vi "Main Loop.vi"(8 "error in (no error)":errorcluster, 10 "Chart Notifier":refnum<notifier>, 11 "Message Queues":T1) -> (0 "error out":errorcluster)   [LabVIEW 2018, in "TCU Module.lvlib" / "TCU Module Engine.lvlib"]
uses:
  TCU Module Engine.lvlib
  All Message Queues.ctl
  support/Message Queue/Message Cluster.ctl
  TCU State Cluster.ctl
  State Enum.ctl
  TCU Module Settings Cluster.ctl
  Output Devices.ctl
  Huber TCU/Huber Settings.ctl
  Lauda Integral XT-150 TCU/Lauda Settings.ctl
  Julabo Type 1 TCU/Julabo Type 1 TCU Folder/Julabo FP-50 Settings.ctl
  Huber Unistat 410 TCU/Huber Unistat 410 RS485 Settings.ctl
  TCU Module Display.ctl
  <vilib>/Platform/TimedLoop/XDataNode/timing_clust.ctl
  <vilib>/Platform/TimedLoop/XDataNode/nitl_modes.ctl
  <vilib>/Platform/TimedLoop/XDataNode/wakeup.ctl
  Tag VIs/Tag FGV Operation Enum.ctl
  TCU Module Config Cluster.ctl
  <vilib>/Utility/miscctls.llb/LVPoint32TypeDef.ctl
  support/Message Queue/Enqueue Message (Single).vi
  <vilib>/Platform/TimedLoop/XDataNode/XDataNode.xnode
  support/Message Queue/Message Queue.lvlib
  <vilib>/Platform/TimedLoop/XDataNode/XDNodeRunTimeDep.lvlib
  TCU Module.lvlib
  Shared Variables/Dynamic Shared Variables.lvlib
  Huber TCU/Huber Ministat 230 TCU.lvlib
  Lauda Integral XT-150 TCU/Lauda TCU.lvlib
  Julabo Type 1 TCU/Julabo Type 1 TCU Folder/Julabo Type FP-50 TCU.lvlib
  support/Support Library.lvlib
  Huber Unistat 410 TCU/Huber Unistat 410 TCU.lvlib
panel:
  out "Period (s)":dbl format="%_4g"
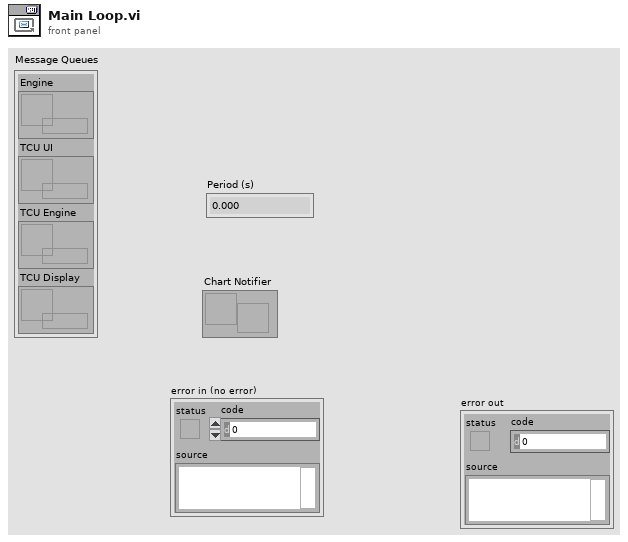
[diagram p1: front panel]
types:
  T1 = typedef "TCU Module.lvlib/All Message Queues.ctl" = cluster{"Engine":refnum<queue>, "TCU UI":refnum<queue>, "TCU Engine":refnum<queue>, "TCU Display":refnum<queue>}
  T2 = typedef "XDNodeRunTimeDep.lvlib/timing_clust.ctl" = cluster{"Expected End [f-1]":u64, "Actual End [f-1]":u64, "Finished Late? [f-1]":bool, "Expected End [i-1]":u64, "Actual End [i-1]":u64, "Finished Late? [i-1]":bool, "Expected Start [i]":u64, "Actual Start [i]":u64, "Expected Start [f]":u64, "Actual Start [f]":u64, "Source Name":string, "Structure Name":string, "Period":i64, "Deadline":i64, "Offset":i64, "Start":i64, "Priority":i32, "Timeout":i32, "Mode":T3, "Wakeup Reason":T4, "Error":errorcluster, "Source Type":string, "Secondary Source Type":string, "Global End Time":u64, "Global Start Time":u64, "Frame Duration":u64, "Iteration Duration":u64, "Assigned CPU":i32, "I/O Scan Engine Mode":u32}
  T3 = typedef "XDNodeRunTimeDep.lvlib/nitl_modes.ctl" = enum32{"No Change", "Process missed periods, maintain original phase", "Discard missed periods, maintain original phase", "Process missed periods, ignore original phase", "Discard missed periods, ignore original phase"}
  T4 = typedef "XDNodeRunTimeDep.lvlib/wakeup.ctl" = enum32{"Normal", "Aborted", "Asynchronous wakeup", "Timing source error", "Timed loop error", "Timeout"}
  T5 = cluster{"enable? (F)":bool, "name":string, "alarm on":bool, "priority":u32, "ack type":enum16{"Auto", "User", "None", "Each Occurrence"}, "area":string, "description":string, "log? (T)":bool}
  T6 = typedef "Tag FGV Operation Enum.ctl" = enum16{"Init", "Set Notification Queue", "Create Tag", "Commit", "Write Tag (Numeric)", "Write Tag (Boolean)", "Read All Tags", "Read One Tag", "Delete Tag Category", "Set Alarm Parameters (Numeric)", "Set Alarm Parameters (Boolean)", "Enable All Alarms", "Disable All Alarms", "Delete All Tags", "Read Alarms", "Ack Alarm", "Read Alarm Parameters (Numeric)", "Read Alarm Parameters (Boolean)"}
  T7 = enum32{"u32BitField", "bool", "double", "string", "int8", "uint8", "int16", "uint16", "int32", "uint32", "int64", "uint64", "single", "double waveform", "int16 waveform", "array of boolean", "array of int8", "array of uint8", "array of int16", "array of uint16", "array of int32", "array of uint32", "array of int64", "array of uint64", "array of single", "array of double", "array of double waveform", "array of int16 waveform", "array of string", "variant", "timestamp", "fixed point", "custom"}
  T8 = typedef "TCU Module.lvlib/TCU Module Engine.lvlib/State Enum.ctl" = enum16{"Measuring", "Idle", "Paused"}
  T9 = typedef "TCU Module.lvlib/TCU Module Config Cluster.ctl" = cluster{"GUID":string, "Drop Coords":T10, "Process Name":string, "User name":string, "Queue Name":string, "Settings":T11, "Load Count":i32, "Power Level Changed":bool}
  T10 = typedef "LVPoint32TypeDef.ctl" = cluster{"Horizontal":i32, "Vertical":i32}
  T11 = typedef "TCU Module.lvlib/TCU Module Settings Cluster.ctl" = cluster{"Cycle Period":dbl, "Setpoint Entry":dbl, "Output Device":T12, "Huber Ministat 230 Settings":T13, "Lauda Settings":T14, "Julabo FP-50 Settings":T15, "Internal Control?":bool, "Huber Unistat 410 Settings":T16}
  T12 = typedef "Output Devices.ctl" = enum16{"Default", "Huber Ministat 230", "Huber Unistat 410", "Lauda XT-150", "Julabo FP-50"}
  T13 = typedef "Huber Ministat 230 TCU.lvlib/Huber Settings.ctl" = cluster{"VISA resource name":refnum<visa-resource-name>, "Simulated?":bool}
  T14 = typedef "Lauda TCU.lvlib/Lauda Settings.ctl" = cluster{"VISA resource name":refnum<visa-resource-name>, "Simulated?":bool, "Pump Power":i32}
  T15 = typedef "Julabo Type FP-50 TCU.lvlib/Julabo FP-50 Settings.ctl" = cluster{"VISA resource name":refnum<visa-resource-name>, "Simulated?":bool, "Pump Power":i32}
  T16 = typedef "Huber Unistat 410 TCU.lvlib/Huber Unistat 410 RS485 Settings.ctl" = cluster{"VISA resource name":refnum<visa-resource-name>, "Address":i8, "Simulated?":bool}
  T17 = typedef "TCU Module.lvlib/TCU Module Display.ctl" = cluster{"TCU On?":bool, "Cycle Period":dbl, "Current TCU Temp":dbl}
  T18 = typedef "TCU Module.lvlib/TCU Module Engine.lvlib/TCU State Cluster.ctl" = cluster{"State":T8, "Start Time":timestamp, "Configuration":T11, "Current Time":timestamp, "First Iteration":bool, "Data":cluster{"TCU Speed":dbl, "Temperature":dbl}, "Process Name":string, "TCU On?":bool, "Output Error":bool, "Start Log":bool, "Power Level Changed":bool}
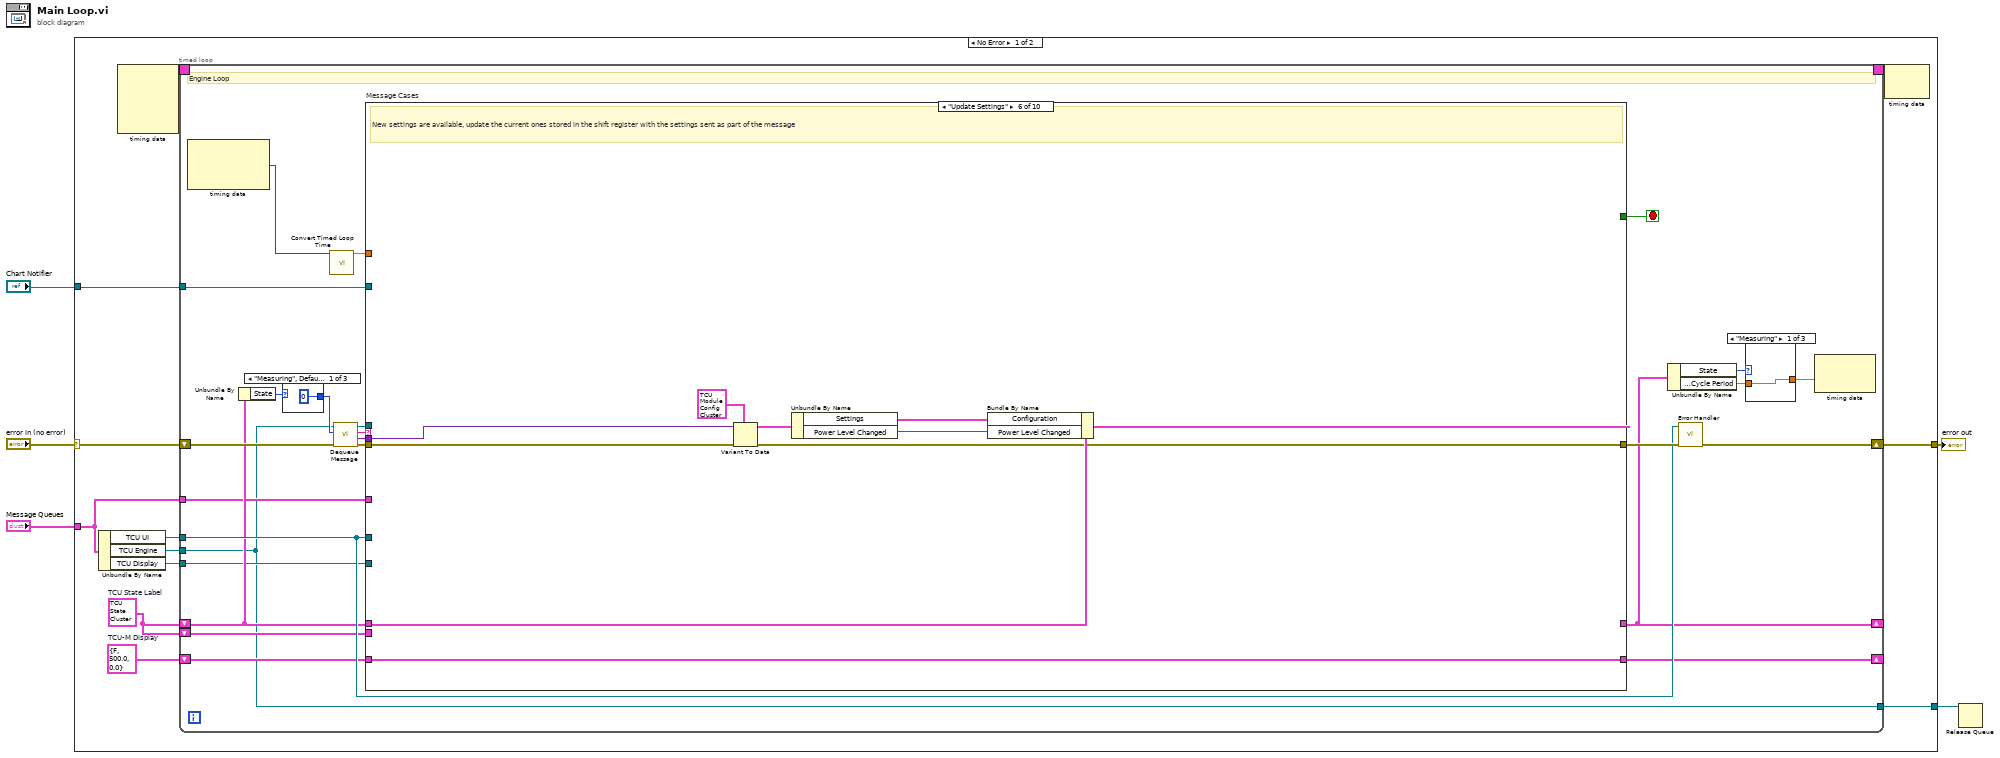
[diagram p0: block diagram]
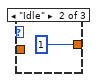
[diagram p2: hidden frame]
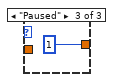
[diagram p3: hidden frame]
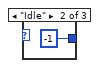
[diagram p4: hidden frame]
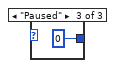
[diagram p5: hidden frame]
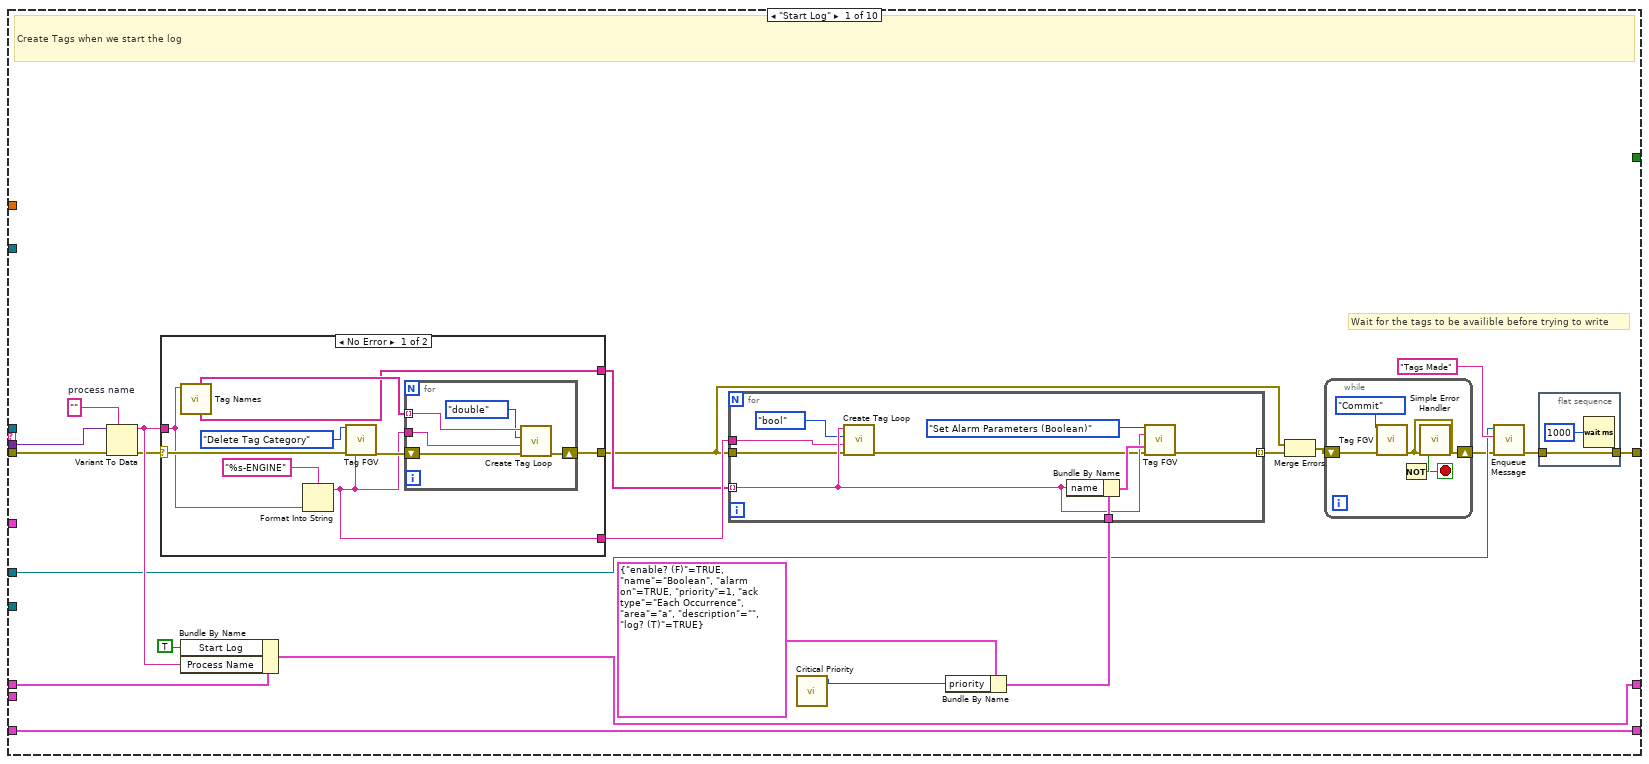
[diagram p6: hidden frame]
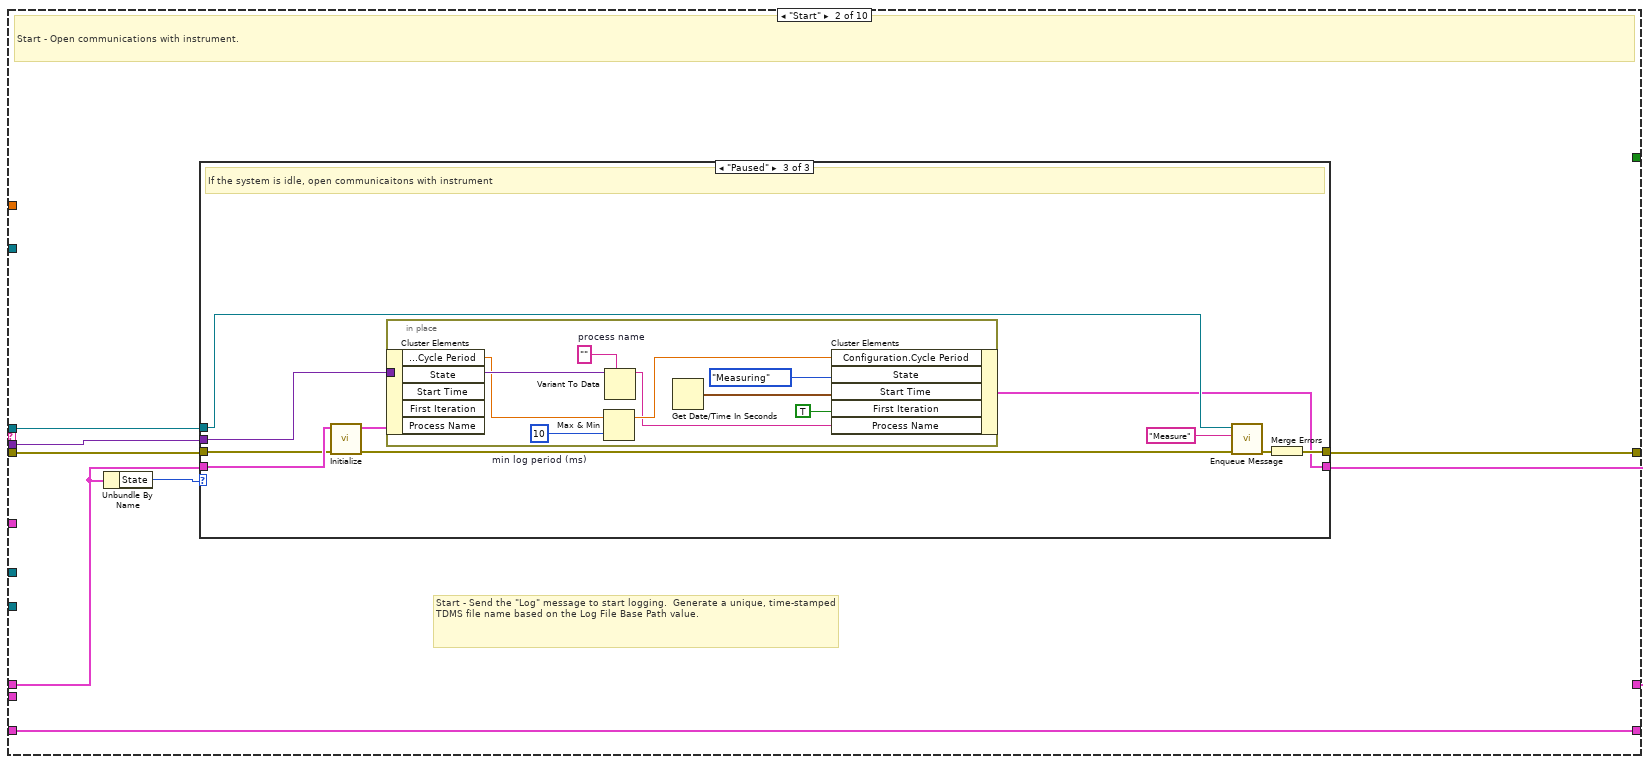
[diagram p8: hidden frame]
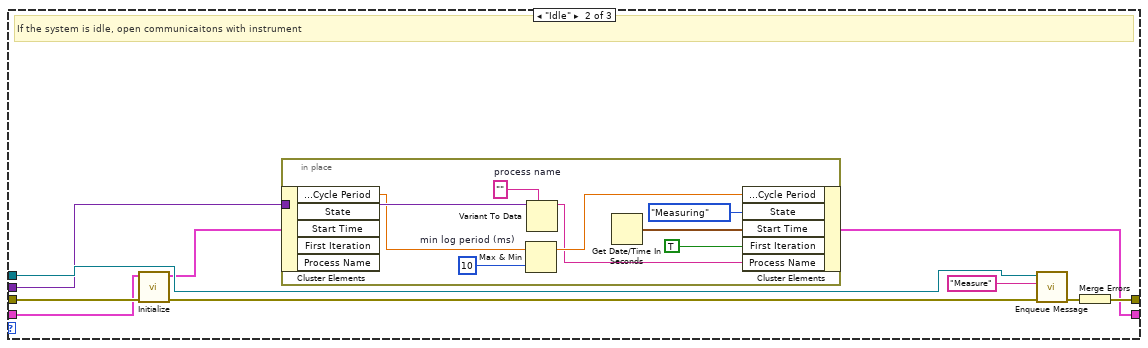
[diagram p10: hidden frame]
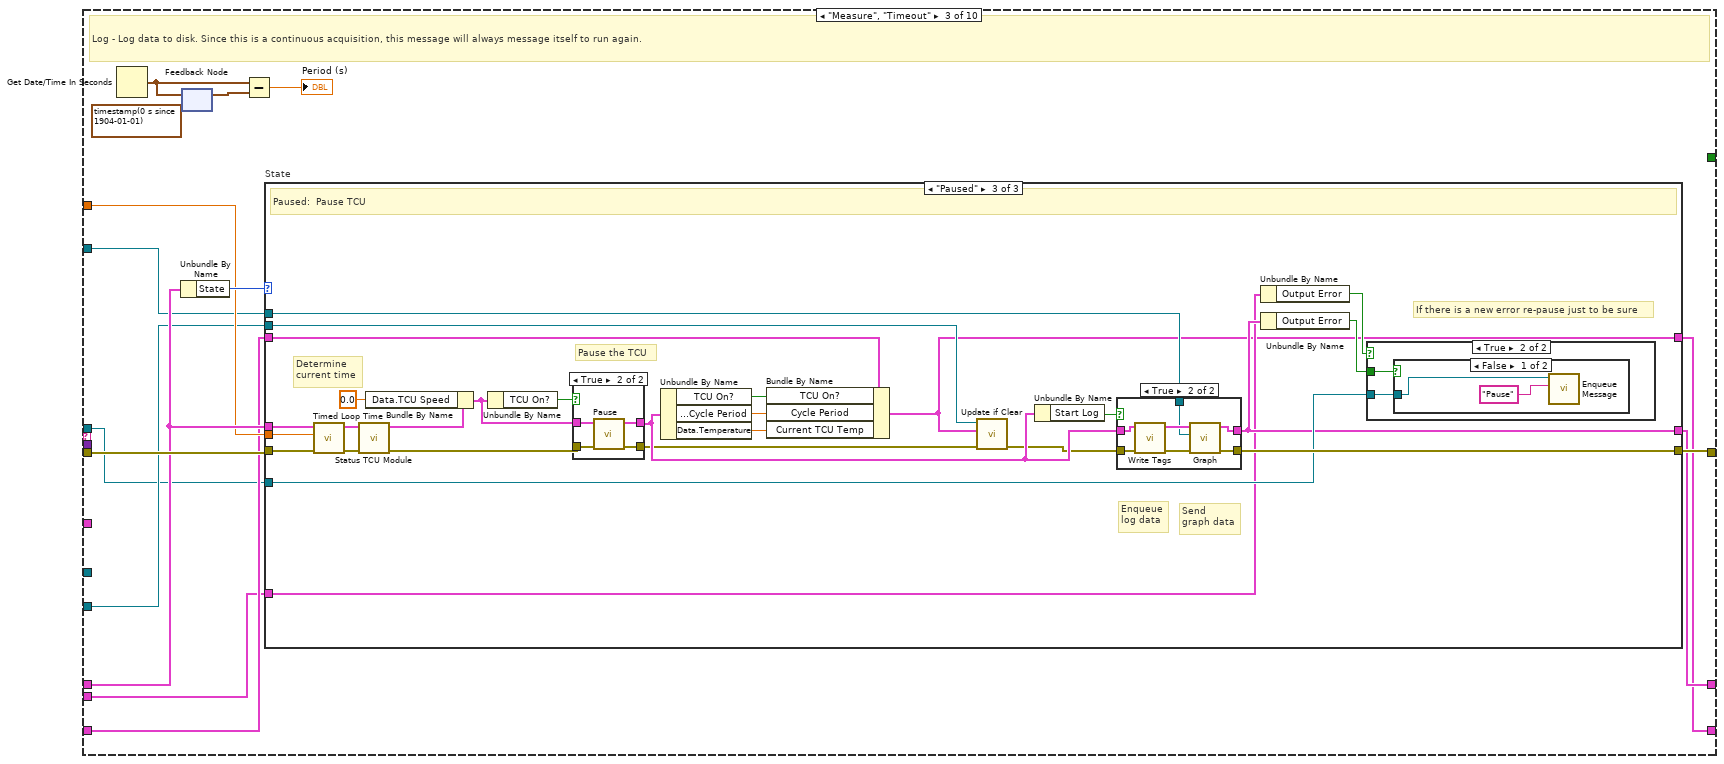
[diagram p11: hidden frame]
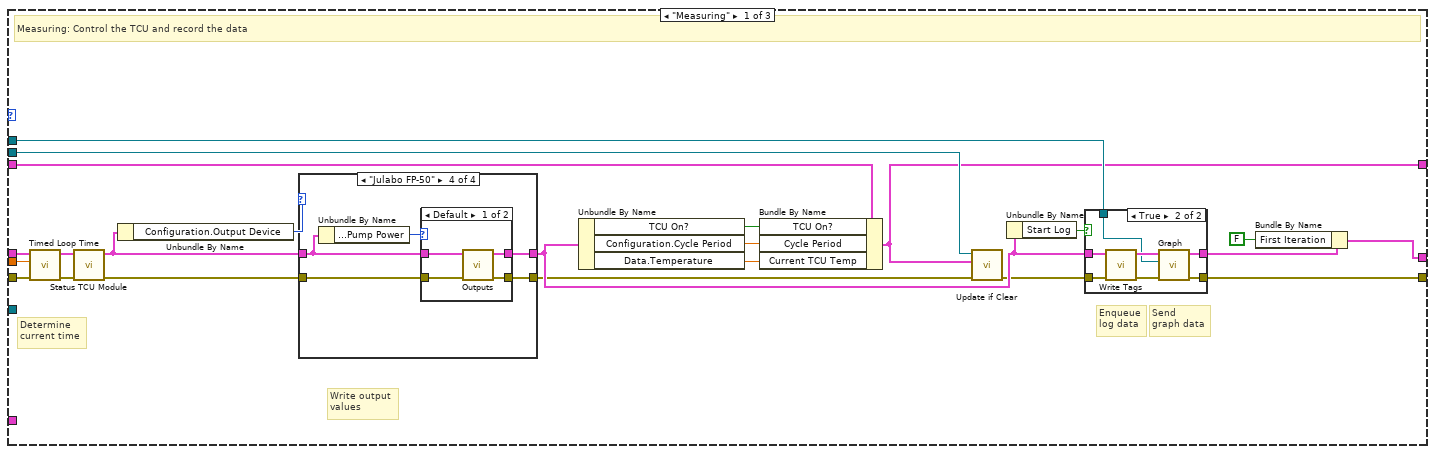
[diagram p12: hidden frame]
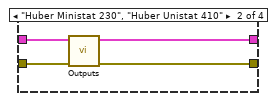
[diagram p14: hidden frame]
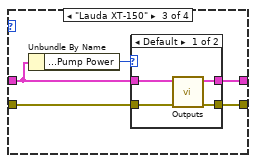
[diagram p15: hidden frame]
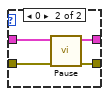
[diagram p16: hidden frame]
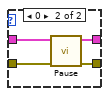
[diagram p17: hidden frame]
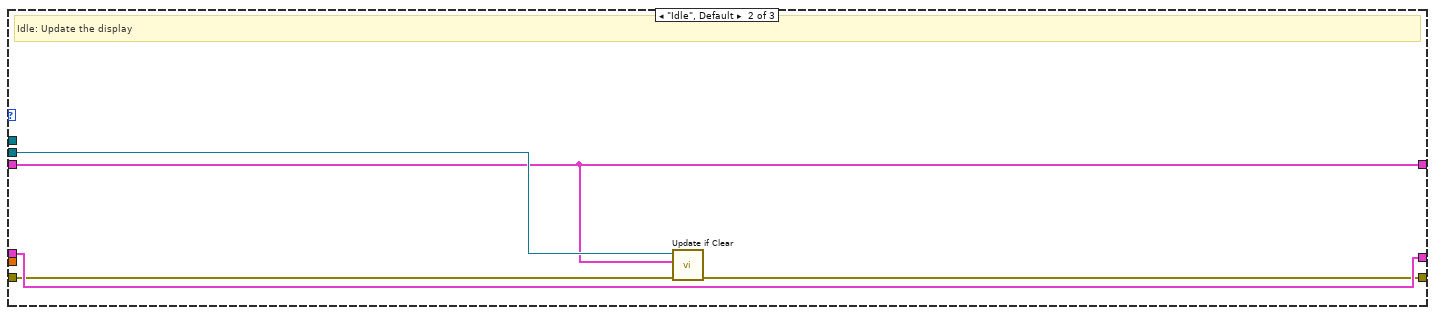
[diagram p19: hidden frame]
diagram:
  n1 = case shown="No Error" "error in (no error)" {
    selector: "error in (no error)" -> [w16 w370]
    tunnel: "Message Queues" -> [w12 _]
    tunnel: [w17 w370] -> w4
    tunnel: "Chart Notifier" -> [w10 _]
    tunnel: [w6 _] -> w1
    frame No Error {
      w8 = T17 {"TCU On?"=FALSE, "Cycle Period"=500.0, "Current TCU Temp"=0.0}  # TCU-M Display
      w7 = T18 {"State"=enum."Idle", "Start Time"=timestamp(0 s since 1904-01-01), "Configuration"={"Cycle Period"=0.0, "Setpoint Entry"=0.0, "Output Device"=enum."Default", "Huber Ministat 230 Settings"={"VISA resource name"="", "Simulated?"=FALSE}, "Lauda Settings"={"VISA resource name"="", "Simulated?"=FALSE, "Pump Power"=2}, "Julabo FP-50 Settings"={"VISA resource name"="", "Simulated?"=FALSE, "Pump Power"=2}, "Internal Control?"=FALSE, "Huber Unistat 410 Settings"={"VISA resource name"="", "Address"=0, "Simulated?"=FALSE}}, "Current Time"=timestamp(0 s since 1904-01-01), "First Iteration"=FALSE, "Data"={"TCU Speed"=0.0, "Temperature"=0.0}, "Process Name"="", "TCU On?"=FALSE, "Output Error"=FALSE, "Start Log"=FALSE, "Power Level Changed"=FALSE}  # TCU State Label
      n2 = Unbundle By Name(w12) -> ("TCU UI"=w15:refnum<queue>, "TCU Engine"=w11:refnum<queue>, "TCU Display"=w9:refnum<queue>)
      n3 = node-c288() -> (w14:T2)  [unwired: 4 in]
      n4 = timed-loop {
        tunnel: w11 -> [w18]
        shift-right: [w30] -> _
        shift-left: w7 -> [w33]
        shift-right: [w35] -> w17
        shift-left: w16 -> [w41]
        tunnel: w15 -> [w34]
        timing: w14 -> [_]
        timing-out: [_] -> w13
        tunnel: w12 -> [w24]
        tunnel: w10 -> [w23]
        tunnel: w9 -> [w22]
        shift-right: [w21] -> _
        shift-left: w8 -> [w20]
        shift-left: w7 -> [w19]
        tunnel: [w18] -> w6
        stop <- w42 stop-if-true
        # "Engine Loop"
        n5 = node-c288() -> (w26:i64)  [unwired: 1 in, 2 out]
        n6 = Unbundle By Name(w33) -> ("State"=w32:T8)
        n7 = case shown="\"Measuring\", Default" w32 {
          tunnel: [0 ("timeout in ms (-1)") -1 ("timeout in ms (-1)") 0 ("timeout in ms (-1)")] -> w31
          frame "Measuring", Default {
          }
          frame "Idle" {
          }
          frame "Paused" {
          }
        }
        n8 = call "Convert Timed Loop Time.vi"("Actual Start [i]"=w26) -> ("ET since start (s)"=w25:dbl)  [unwired: 10 in]
        n9 = call "Dequeue Message.vi"("error in (no error)"=w41, "timeout in ms (-1)"=w31, "Message Queue"=w18) -> ("error out"=w40:errorcluster, "Message Data"=w38:variant, "Message"=w39:string, "dup Message Queue"=w37:refnum<queue>)  [unwired: 5 in]
        n10 = case "Message Cases" shown="\"Update Settings\"" w39 {
          selector: w39 -> [_ _ _ _ _ _ _ _ _ w360]
          tunnel: w37 -> [_ w113 w157 _ _ _ w342 _ _ _]
          tunnel: w40 -> [w73 w112 w168 w294 w313 w336 w345 w352 w359 _]
          tunnel: [w55 w114 w169 w286 w306 w332 w347 w350 w358 w361] -> w36
          tunnel: w33 -> [w72 w108 w166 w291 w311 w334 w340 w351 w356 w367]
          tunnel: [w71 w111 w167 w290 w310 w333 w340 w351 w353 w367] -> w30
          tunnel: [_ _ _ _ _ _ TRUE _ _ _] -> w42
          tunnel: w38 -> [w74 w109 _ _ _ w337 _ _ _ _]
          tunnel: w34 -> [w59 _ _ w293 _ _ w346 _ _ _]
          tunnel: w25 -> [_ _ w165 _ _ _ _ _ _ _]
          tunnel: w24 -> [_ _ _ _ _ _ _ _ _ _]
          tunnel: w23 -> [_ _ w161 _ _ _ _ _ _ _]
          tunnel: w22 -> [_ _ w160 w289 w309 _ _ _ _ _]
          tunnel: w20 -> [w75 w107 w159 w288 w308 w335 w338 w349 w357 w366]
          tunnel: [w75 w107 w158 w288 w308 w335 w338 w349 w357 w366] -> w21
          tunnel: w19 -> [_ _ w156 _ _ _ _ _ _ _]
          frame "Start Log" {
            w70 = ""  # process name
            # "Wait for the tags to be availible before trying to write"
            # "Create Tags when we start the log"
            n11 = Variant To Data(error in=w73, type=w70, Variant=w74) -> (data=w69:string, error out=w68:errorcluster)
            n12 = case shown="No Error" w68 {
              selector: w68 -> [w97 w106]
              tunnel: [w100 w106] -> w54
              tunnel: w69 -> [w95 _]
              tunnel: [w93 _] -> w64
              tunnel: [w92 _] -> w63
              frame No Error {
                n13 = call "Tag Names.vi"("Process Name"=w95) -> ("All Boolean Tags"=w92:string[], "All  Numeric Tags"=w94:string[])  [unwired: 8 in, 1 out]
                n14 = Format Into String(format string="%s-ENGINE", w95) -> (resulting string=w93:string)  [unwired: 2 in, 1 out]
                n15 = call "Tag FGV.vi"("Operation"=Tag_FGV_Operation_Enum."Delete Tag Category", "error in (no error)"=w97, "Tag Category"=w93) -> ("error out"=w96:errorcluster)  [unwired: 5 in, 7 out]
                n16 = for {
                  shift-right: [w101] -> w100
                  shift-left: w96 -> [w104]
                  tunnel: w93 -> [w103]
                  tunnel: w94 -> [w105] mode=indexing
                  n17 = call "Create Tag Loop.vi"("error in (no error)"=w104, "Tag Category"=w103, "data type"=T7."double", "Tag Name"=w105) -> ("error out"=w101:errorcluster)  [unwired: 7 in]
                }
              }
              frame Error {
              }
            }
            n18 = Bundle By Name(cluster=w72, "Start Log"=TRUE, "Process Name"=w69) -> (w71:T18)
            n19 = call "Critical Priority.vi"() -> ("critical priority"=w67:i32)  [unwired: 11 in]
            n20 = Bundle By Name(cluster=T5 {"enable? (F)"=TRUE, "name"="Boolean", "alarm on"=TRUE, "priority"=1, "ack type"=enum."Each Occurrence", "area"="a", "description"="", "log? (T)"=TRUE} ("Boolean alarm settings"), "priority"=w67) -> (w65:T5)
            n21 = for {
              tunnel: w65 -> [w91]
              tunnel: [w90] -> w62 mode=indexing
              tunnel: w63 -> [w87] mode=indexing
              tunnel: w54 -> [w84]
              tunnel: w64 -> [w85]
              n22 = call "Create Tag Loop.vi"("error in (no error)"=w84, "Tag Category"=w85, "data type"=T7."bool", "Tag Name"=w87) -> ("error out"=w83:errorcluster)  [unwired: 7 in]
              n23 = Bundle By Name(cluster=w91, "name"=w87) -> (w89:T5)
              n24 = call "Tag FGV.vi"("Operation"=Tag_FGV_Operation_Enum."Set Alarm Parameters (Boolean)", "Tag Name"=w87, "Data"=w89, "error in (no error)"=w83) -> ("error out"=w90:errorcluster)  [unwired: 4 in, 7 out]
            }
            n25 = Merge Errors(w54, w62) -> (w58:errorcluster)
            n26 = while {
              shift-right: [w80] -> w57
              shift-left: w58 -> [w81]
              stop <- w78 stop-if-true
              n27 = call "Tag FGV.vi"("Operation"=Tag_FGV_Operation_Enum."Commit", "error in (no error)"=w81) -> ("error out"=w80:errorcluster)  [unwired: 6 in, 7 out]
              n28 = call <vilib>:"Simple Error Handler.vi"("error in (no error)"=w80) -> ("error?"=w79:bool)  [unwired: 4 in, 4 out]
              n29 = Not(x=w79) -> (.not. x?=w78:bool)
            }
            n30 = call-poly "Enqueue Message.vi"("error in (no error)"=w57, "Message"="Tags Made", "Message Queue"=w59) -> ("error out"=w56:errorcluster)  [unwired: 7 in, 1 out]
            n31 = flat-sequence {
              tunnel: w56 -> [w76]
              tunnel: [w76] -> w55
              frame #0 {
                n32 = Wait (ms)(milliseconds to wait=u32 1000) -> ()  [unwired: 1 out]
              }
            }
          }
          frame "Start" {
            # "Start - Send the \"Log\" message to start logging.  Generate a unique, time-stamped TDMS file name based on the Log File Base Path value."
            # "Start - Open communications with instrument."
            n33 = Unbundle By Name(w108) -> ("State"=w110:T8)
            n34 = case shown="\"Paused\"" w110 {
              tunnel: [w115 w126 w145] -> w114
              tunnel: w113 -> [_ w123 w142]
              tunnel: w112 -> [w115 w122 w139]
              tunnel: w108 -> [w116 w121 w140]
              tunnel: [w116 w117 w136] -> w111
              tunnel: w109 -> [_ w120 w141]
              frame "Measuring", Default {
                # "The system is already running. Ignore the \"Start\" message."
              }
              frame "Idle" {
                # "If the system is idle, open communicaitons with instrument"
                n35 = call "Initialize.vi"("error in (no error)"=w122, "State in"=w121) -> ("error out"=w119:errorcluster, "State out"=w118:T18)  [unwired: 8 in]
                n36 = in-place {
                  in-place-border: w120 -> [w133]
                  w134 = ""  # process name
                  w135 = 10  # min log period (ms)
                  n37 = in-place-cluster #1(w118) -> ("Configuration.Cycle Period"=w132:dbl)  [unwired: 4 out]
                  n38 = Max & Min(x=w132, y=w135) -> (max(x,y)=w131:dbl)  [unwired: 1 out]
                  n39 = Variant To Data(type=w134, Variant=w133) -> (data=w127:string)  [unwired: 1 in, 1 out]
                  n40 = Get Date/Time In Seconds() -> (seconds since 1Jan1904=w129:timestamp)
                  n41 = in-place-cluster #1("Configuration.Cycle Period"=w131, "State"=State_Enum."Measuring", "Start Time"=w129, "First Iteration"=TRUE, "Process Name"=w127) -> (w117:T18)
                }
                n42 = call-poly "Enqueue Message.vi"("error in (no error)"=w119, "Message"="Measure", "Message Queue"=w123) -> ("error out"=w124:errorcluster)  [unwired: 7 in, 1 out]
                n43 = Merge Errors(w124) -> (w126:errorcluster)
              }
              frame "Paused" {
                # "If the system is idle, open communicaitons with instrument"
                n44 = call "Initialize.vi"("error in (no error)"=w139, "State in"=w140) -> ("error out"=w138:errorcluster, "State out"=w137:T18)  [unwired: 8 in]
                n45 = in-place {
                  in-place-border: w141 -> [w152]
                  w153 = ""  # process name
                  w154 = 10  # min log period (ms)
                  n46 = in-place-cluster #2(w137) -> ("Configuration.Cycle Period"=w151:dbl)  [unwired: 4 out]
                  n47 = Max & Min(x=w151, y=w154) -> (max(x,y)=w150:dbl)  [unwired: 1 out]
                  n48 = Variant To Data(type=w153, Variant=w152) -> (data=w146:string)  [unwired: 1 in, 1 out]
                  n49 = Get Date/Time In Seconds() -> (seconds since 1Jan1904=w148:timestamp)
                  n50 = in-place-cluster #2("Configuration.Cycle Period"=w150, "State"=State_Enum."Measuring", "Start Time"=w148, "First Iteration"=TRUE, "Process Name"=w146) -> (w136:T18)
                }
                n51 = call-poly "Enqueue Message.vi"("error in (no error)"=w138, "Message"="Measure", "Message Queue"=w142) -> ("error out"=w143:errorcluster)  [unwired: 7 in, 1 out]
                n52 = Merge Errors(w143) -> (w145:errorcluster)
              }
            }
          }
          frame "Measure", "Timeout" {
            # "Log - Log data to disk. Since this is a continuous acquisition, this message will always message itself to run again."
            n53 = Get Date/Time In Seconds() -> (seconds since 1Jan1904=w163:timestamp)
            n54 = Unbundle By Name(w166) -> ("State"=w170:T8)
            n55 = feedback-in #3(w163) -> ()
            n56 = feedback #3(timestamp(0 s since 1904-01-01) ("seconds since 1Jan1904")) -> (w164:timestamp)
            n57 = Subtract(x=w163, y=w164) -> (x-y=→"Period (s)":dbl)
            n58 = case "State" shown="\"Paused\"" w170 {
              tunnel: w168 -> [w192 w236 w262]
              tunnel: w166 -> [w191 w239 w263]
              tunnel: [w193 w235 w258] -> w169
              tunnel: [w188 w239 w253] -> w167
              tunnel: w165 -> [w190 _ w265]
              tunnel: w161 -> [w186 _ w266]
              tunnel: w160 -> [w174 w238 w243]
              tunnel: w159 -> [w185 w237 w264]
              tunnel: [w173 w237 w242] -> w158
              tunnel: w157 -> [_ _ w254]
              tunnel: w156 -> [_ _ w250]
              frame "Measuring" {
                # "Determine\ncurrent time"
                # "Send\ngraph data"
                # "Enqueue\nlog data"
                # "Write output\nvalues"
                # "Measuring: Control the TCU and record the data"
                n59 = call "Timed Loop Time.vi"("error in (no error)"=w192, "ET since start (s)"=w190, "State in"=w191) -> ("error out"=w183:errorcluster, "State out"=w182:T18)  [unwired: 7 in]
                n60 = call "Status TCU Module.vi"("error in (no error)"=w183, 11:w182) -> ("error out"=w176:errorcluster, "State out"=w177:T18)  [unwired: 8 in]
                n61 = Unbundle By Name(w177) -> ("Configuration.Output Device"=w178:T12)
                n62 = case shown="\"Julabo FP-50\"" w178 {
                  tunnel: w177 -> [w195 w199 w204 w216]
                  tunnel: w176 -> [w194 w198 w201 w215]
                  tunnel: [w195 w196 w202 w213] -> w175
                  tunnel: [w194 w197 w203 w214] -> w172
                  frame Default {
                  }
                  frame "Huber Ministat 230", "Huber Unistat 410" {
                    n63 = call "Outputs.vi"("error in (no error)"=w198, "State in"=w199) -> ("error out"=w197:errorcluster, "State out"=w196:T18)  [unwired: 8 in]
                  }
                  frame "Lauda XT-150" {
                    n64 = Unbundle By Name(w204) -> ("Configuration.Lauda Settings.Pump Power"=w200:i32)
                    n65 = case shown="Default" w200 {
                      tunnel: w201 -> [w208 w211]
                      tunnel: [w207 w210] -> w203
                      tunnel: w204 -> [w206 w212]
                      tunnel: [w205 w209] -> w202
                      frame Default {
                        n66 = call "Outputs.vi"("error in (no error)"=w208, "State in"=w206) -> ("error out"=w207:errorcluster, "State out"=w205:T18)  [unwired: 8 in]
                      }
                      frame 0 {
                        n67 = call "Pause.vi"("error in (no error)"=w211, "State in"=w212) -> ("error out"=w210:errorcluster, "State out"=w209:T18)  [unwired: 8 in]
                      }
                    }
                  }
                  frame "Julabo FP-50" {
                    n68 = Unbundle By Name(w216) -> ("Configuration.Julabo FP-50 Settings.Pump Power"=w217:i32)
                    n69 = case shown="Default" w217 {
                      tunnel: w215 -> [w221 w224]
                      tunnel: [w220 w223] -> w214
                      tunnel: w216 -> [w219 w225]
                      tunnel: [w218 w222] -> w213
                      frame Default {
                        n70 = call "Outputs.vi"("error in (no error)"=w221, "State in"=w219) -> ("error out"=w220:errorcluster, "State out"=w218:T18)  [unwired: 8 in]
                      }
                      frame 0 {
                        n71 = call "Pause.vi"("error in (no error)"=w224, "State in"=w225) -> ("error out"=w223:errorcluster, "State out"=w222:T18)  [unwired: 8 in]
                      }
                    }
                  }
                }
                n72 = Unbundle By Name(w175) -> ("TCU On?"=w184:bool, "Configuration.Cycle Period"=w181:dbl, "Data.Temperature"=w180:dbl)
                n73 = Bundle By Name(cluster=w185, "TCU On?"=w184, "Cycle Period"=w181, "Current TCU Temp"=w180) -> (w173:T17)
                n74 = call "Update if Clear.vi"("error in (no error)"=w172, "Message Data"=w173, "Queue in"=w174) -> ("error out"=w171:errorcluster)  [unwired: 8 in]
                n75 = Unbundle By Name(w175) -> ("Start Log"=w179:bool)
                n76 = case shown="True" w179 {
                  tunnel: [w226 w232] -> w193
                  tunnel: [w227 w231] -> w189
                  tunnel: w186 -> [_ w230]
                  tunnel: w175 -> [w227 w229]
                  tunnel: w171 -> [w226 w228]
                  frame False {
                  }
                  frame True {
                    n77 = call "Write Tags.vi"("error in (no error)"=w228, "State in"=w229) -> ("error out"=w233:errorcluster, "State out"=w234:T18)  [unwired: 8 in]
                    n78 = call "Graph.vi"("error in (no error)"=w233, "notifier out"=w230, "State in"=w234) -> ("error out"=w232:errorcluster, "State out"=w231:T18)  [unwired: 7 in]
                  }
                }
                n79 = Bundle By Name(cluster=w189, "First Iteration"=FALSE) -> (w188:T18)
              }
              frame "Idle", Default {
                # "Idle: Update the display"
                n80 = call "Update if Clear.vi"("error in (no error)"=w236, "Message Data"=w237, "Queue in"=w238) -> ("error out"=w235:errorcluster)  [unwired: 8 in]
              }
              frame "Paused" {
                # "If there is a new error re-pause just to be sure"
                # "Determine\ncurrent time"
                # "Pause the TCU"
                # "Send\ngraph data"
                # "Enqueue\nlog data"
                # "Paused:  Pause TCU"
                n81 = call "Timed Loop Time.vi"("error in (no error)"=w262, "ET since start (s)"=w265, "State in"=w263) -> ("error out"=w260:errorcluster, "State out"=w261:T18)  [unwired: 7 in]
                n82 = call "Status TCU Module.vi"("error in (no error)"=w260, 11:w261) -> ("error out"=w259:errorcluster, "State out"=w246:T18)  [unwired: 8 in]
                n83 = Bundle By Name(cluster=w246, "Data.TCU Speed"=0.0) -> (w244:T18)
                n84 = Unbundle By Name(w244) -> ("TCU On?"=w247:bool)
                n85 = case shown="True" w247 {
                  tunnel: w244 -> [w277 w281]
                  tunnel: w259 -> [w276 w280]
                  tunnel: [w276 w279] -> w241
                  tunnel: [w277 w278] -> w249
                  frame False {
                  }
                  frame True {
                    n86 = call "Pause.vi"("error in (no error)"=w280, "State in"=w281) -> ("error out"=w279:errorcluster, "State out"=w278:T18)  [unwired: 8 in]
                  }
                }
                n87 = Unbundle By Name(w249) -> ("TCU On?"=w257:bool, "Configuration.Cycle Period"=w256:dbl, "Data.Temperature"=w255:dbl)
                n88 = Bundle By Name(cluster=w264, "TCU On?"=w257, "Cycle Period"=w256, "Current TCU Temp"=w255) -> (w242:T17)
                n89 = call "Update if Clear.vi"("error in (no error)"=w241, "Message Data"=w242, "Queue in"=w243) -> ("error out"=w240:errorcluster)  [unwired: 8 in]
                n90 = Unbundle By Name(w249) -> ("Start Log"=w248:bool)
                n91 = case shown="True" w248 {
                  tunnel: w266 -> [_ w273]
                  tunnel: w240 -> [w267 w272]
                  tunnel: [w267 w271] -> w258
                  tunnel: w249 -> [w268 w270]
                  tunnel: [w268 w269] -> w253
                  frame False {
                  }
                  frame True {
                    n92 = call "Write Tags.vi"("error in (no error)"=w272, "State in"=w270) -> ("error out"=w275:errorcluster, "State out"=w274:T18)  [unwired: 8 in]
                    n93 = call "Graph.vi"("error in (no error)"=w275, "notifier out"=w273, "State in"=w274) -> ("error out"=w271:errorcluster, "State out"=w269:T18)  [unwired: 7 in]
                  }
                }
                n94 = Unbundle By Name(w250) -> ("Output Error"=w251:bool)
                n95 = Unbundle By Name(w253) -> ("Output Error"=w252:bool)
                n96 = case shown="True" w251 {
                  tunnel: w252 -> [_ w283]
                  tunnel: w254 -> [_ w282]
                  frame False {
                  }
                  frame True {
                    n97 = case shown="False" w283 {
                      tunnel: w282 -> [w285 _]
                      frame False {
                        n98 = call-poly "Enqueue Message.vi"("Message"="Pause", "Message Queue"=w285) -> ()  [unwired: 8 in, 2 out]
                      }
                      frame True {
                      }
                    }
                  }
                }
              }
            }
          }
          frame "Stop" {
            # "Stop - Stop the TCU and Close the Connections"
            n99 = Unbundle By Name(w291) -> ("State"=w292:T8)
            n100 = case shown="\"Measuring\", Default" w292 {
              tunnel: [w299 w305] -> w287
              tunnel: w294 -> [w296 w305]
              tunnel: w293 -> [w303 _]
              tunnel: w291 -> [w297 w304]
              tunnel: [w301 w304] -> w290
              frame "Measuring", Default {
                # "If the system is logging, stop logging."
                n101 = call "Close.vi"("error in (no error)"=w296, "State in"=w297) -> ("error out"=w295:errorcluster, "State out"=w298:T18)  [unwired: 8 in]
                n102 = Bundle By Name(cluster=w298, "State"=State_Enum."Idle") -> (w301:T18)
                n103 = call-poly "Enqueue Message.vi"("error in (no error)"=w295, "Message"="Logging Stopped", "Message Queue"=w303) -> ("error out"=w299:errorcluster)  [unwired: 7 in, 1 out]
              }
              frame "Idle" {
                # "The system is already idle. Ignore the \"Stop\" message."
              }
            }
            n104 = call "Update if Clear.vi"("error in (no error)"=w287, "Message Data"=w288, "Queue in"=w289) -> ("error out"=w286:errorcluster)  [unwired: 8 in]
          }
          frame "Pause" {
            # "Pause: Stop the TCU but don't disconnect"
            n105 = Unbundle By Name(w311) -> ("State"=w312:T8)
            n106 = case shown="\"Measuring\", Default" w312 {
              tunnel: [w318 w320 w327] -> w307
              tunnel: w313 -> [w316 w320 w327]
              tunnel: w311 -> [w317 w321 w325]
              tunnel: [w314 w322 w324] -> w310
              frame "Measuring", Default {
                # "If the system is logging, stop logging."
                n107 = call "Pause.vi"("error in (no error)"=w316, "State in"=w317) -> ("error out"=w318:errorcluster, "State out"=w315:T18)  [unwired: 8 in]
                n108 = Bundle By Name(cluster=w315, "State"=State_Enum."Paused") -> (w314:T18)
              }
              frame "Idle" {
                # "The system is already idle. Ignore the \"Stop\" message."
                n109 = Bundle By Name(cluster=w321, "State"=State_Enum."Paused") -> (w322:T18)
              }
              frame "Paused" {
                n110 = Bundle By Name(cluster=w325, "State"=State_Enum."Paused") -> (w324:T18)
              }
            }
            n111 = call "Update if Clear.vi"("error in (no error)"=w307, "Message Data"=w308, "Queue in"=w309) -> ("error out"=w306:errorcluster)  [unwired: 8 in]
          }
          frame "Update Settings" {
            # "New settings are available, update the current ones stored in the shift register with the settings sent as part of the message"
            n112 = Variant To Data(error in=w336, type=T9 {"GUID"="", "Drop Coords"={"Horizontal"=0, "Vertical"=0}, "Process Name"="", "User name"="", "Queue Name"="", "Settings"={"Cycle Period"=0.0, "Setpoint Entry"=0.0, "Output Device"=enum."Default", "Huber Ministat 230 Settings"={"VISA resource name"="", "Simulated?"=FALSE}, "Lauda Settings"={"VISA resource name"="", "Simulated?"=FALSE, "Pump Power"=2}, "Julabo FP-50 Settings"={"VISA resource name"="", "Simulated?"=FALSE, "Pump Power"=2}, "Internal Control?"=FALSE, "Huber Unistat 410 Settings"={"VISA resource name"="", "Address"=0, "Simulated?"=FALSE}}, "Load Count"=0, "Power Level Changed"=FALSE} ("TCU Module Config Out"), Variant=w337) -> (data=w330:T9, error out=w332:errorcluster)
            n113 = Unbundle By Name(w330) -> ("Settings"=w328:T11, "Power Level Changed"=w329:bool)
            n114 = Bundle By Name(cluster=w334, "Configuration"=w328, "Power Level Changed"=w329) -> (w333:T18)
          }
          frame "Exit" {
            # "Release the Logging queue reference"
            # "Don't check the error out. The UI message queue may have already been released."
            # "Stop the VI"
            # "Exit - Send the Exit message to the UI Message Handler.  Call 'Flush Data to Log File.vi' so any pending data is not lost."
            n115 = Release Queue(queue=w342, error in (no error)=w345) -> (error out=w341:errorcluster)  [unwired: 1 in, 2 out]
            n116 = call-poly "Enqueue Message.vi"("Priority Message? (F)"=TRUE, "Message"="Exit", "Message Queue"=w346) -> ("error out"=w339:errorcluster)  [unwired: 7 in, 1 out]
            n117 = call <vilib>:"Clear Errors.vi"("error in (no error)"=w339) -> ()  [unwired: 5 in, 2 out]
            n118 = Merge Errors(w341) -> (w347:errorcluster)
          }
          frame "---Copy This Frame---" {
            # "Duplicate this frame when creating new messages.  Change this comment in the duplicated frame to describe this message."
            n119 = Merge Errors(w352) -> (w350:errorcluster)
          }
          frame "Initialize" {
            # "Reset First Iteration and Start Log"
            n120 = Merge Errors(w359) -> (w358:errorcluster)
            n121 = Bundle By Name(cluster=w356, "First Iteration"=TRUE, "Start Log"=FALSE) -> (w353:T18)
          }
          frame Default {
            # "'Default' case only runs if there is a message that isn't defined in any of the other cases.  Output a programming error."
            n122 = Concatenate Strings("The invalid message string " ("string"), w360, " was received in the TCU Module Engine." ("string")) -> (w362:string)
            n123 = Bundle By Name(cluster=errorcluster {"status"=TRUE, "code"=1, "source"=""} ("error constant"), "source"=w362) -> (w361:errorcluster)
          }
        }
        n124 = Unbundle By Name(w30) -> ("State"=w29:T8, "Configuration.Cycle Period"=w27:dbl)
        n125 = call "Error Handler.vi"("error in (no error)"=w36, "Message Queue"=w34) -> ("dup error in"=w35:errorcluster)  [unwired: 8 in, 1 out]
        n126 = case shown="\"Measuring\"" w29 {
          tunnel: [w43 1 1] -> w28
          tunnel: w27 -> [w43 _ _]
          frame "Measuring" {
          }
          frame "Idle" {
          }
          frame "Paused" {
          }
        }
        n127 = node-c288(w28) -> ()  [unwired: 1 in, 1 out]
      }
      n128 = node-c288(w13) -> ()  [unwired: 1 out]
    }
    frame Error {
    }
  }
  "error out" <- w4
  n129 = Release Queue(queue=w1) -> ()  [unwired: 2 in, 3 out]
